vi "getRfStateByName.vi"(8 "error in (no error)":errorcluster, 10 "stateName":string, 11 "rf in":refnum<class "rf.lvclass">) -> (0 "error out":errorcluster, 1 "phase":dbl, 2 "frequency":dbl, 3 "rf out":refnum<class "rf.lvclass">)   [LabVIEW 2011, in "Tools.lvlib" / "Scripting.lvlib" / "rf.lvclass"]
uses:
  rf.lvclass
  DatabaseHelpers/Database Objects/Channel/RfOutputChannel/RfOutputChannel.lvclass
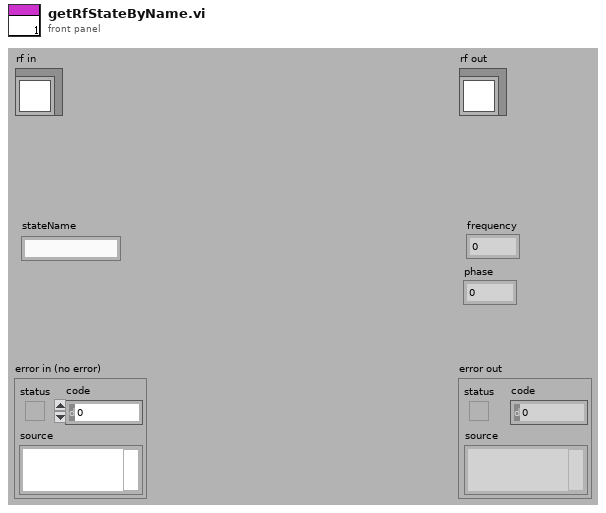
[diagram p1: front panel]
types:
  T1 = cluster{"state_name":string, "value":cluster{"frequency":string, "amplitude":string, "phase":string}}[]
  T2 = cluster{"state_name":string, "value":cluster{"frequency":string, "amplitude":string, "phase":string}}
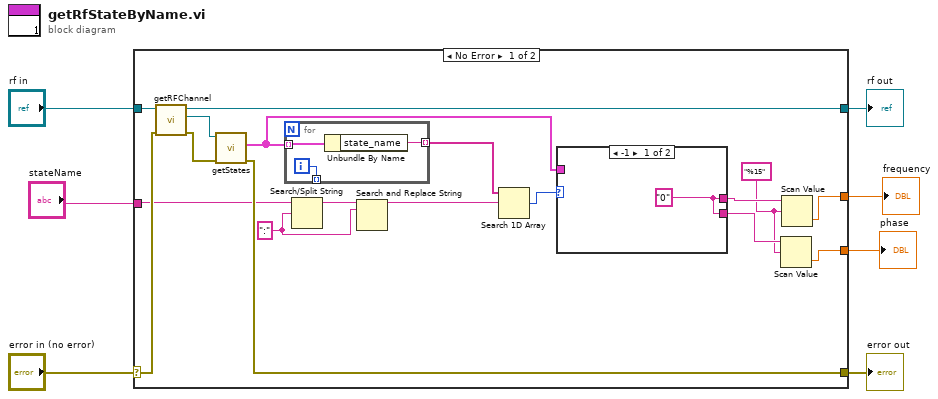
[diagram p0: block diagram]
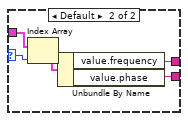
[diagram p2: hidden frame]
diagram:
  n1 = case shown="No Error" "error in (no error)" {
    selector: "error in (no error)" -> [w24 w36]
    tunnel: [w12 w36] -> w6
    tunnel: [w22 w35] -> w4
    tunnel: "rf in" -> [w25 w35]
    tunnel: "stateName" -> [w11 _]
    tunnel: [w16 _] -> w2
    tunnel: [w14 _] -> w1
    frame No Error {
      w10 = ":"
      w13 = "%15" ("format string")
      n2 = call "getRFChannel.vi"("error in (no error)"=w24, "rf.lvclass in"=w25) -> ("error out"=w23:errorcluster, "RfOutputChannel.lvclass"=w21:refnum<class "RfOutputChannel.lvclass">, "rf.lvclass out"=w22:refnum<class "rf.lvclass">)  [unwired: 7 in]
      n3 = call "getStates.vi"("error in (no error)"=w23, "RfOutputChannel in"=w21) -> ("error out"=w12:errorcluster, "states"=w18:T1)  [unwired: 7 in, 1 out]
      n4 = for {
        tunnel: w18 -> [w34] mode=indexing
        tunnel: [w33] -> w20 mode=indexing
        tunnel: [w32] -> _ mode=indexing
        i -> [w32]
        n5 = Unbundle By Name(w34) -> ("state_name"=w33:string)
      }
      n6 = Search/Split String(string=w11, search string/char (-)=w10) -> (substring before match=w8:string)  [unwired: 1 in, 2 out]
      n7 = Search and Replace String(input string=w8, search string=w10) -> (result string=w9:string)  [unwired: 6 in, 3 out]
      n8 = Search 1D Array(1D array=w20, element=w9) -> (index of element=w19:i32)  [unwired: 1 in]
      n9 = case shown="-1" w19 {
        selector: w19 -> [_ w31]
        tunnel: w18 -> [_ w30]
        tunnel: [w26 w28] -> w17
        tunnel: [w26 w27] -> w15
        frame -1 {
          w26 = "0"
        }
        frame Default {
          n10 = Index Array(array=w30, index=w31) -> (element=w29:T2)
          n11 = Unbundle By Name(w29) -> ("value.frequency"=w28:string, "value.phase"=w27:string)
        }
      }
      n12 = Scan Value(string=w15, format string=w13) -> (value=w14:dbl)  [unwired: 1 in, 1 out]
      n13 = Scan Value(string=w17, format string=w13) -> (value=w16:dbl)  [unwired: 1 in, 1 out]
    }
    frame Error {
    }
  }
  "error out" <- w6
  "rf out" <- w4
  "frequency" <- w2
  "phase" <- w1
